vi "VVERFT.vi"(1 "Vector":dbl[](array[numeric])) -> (0 "Funcion de transferencia":string)   [LabVIEW 2019]
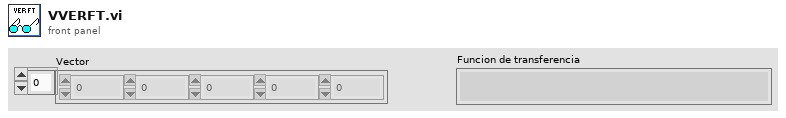
[diagram p1: front panel]
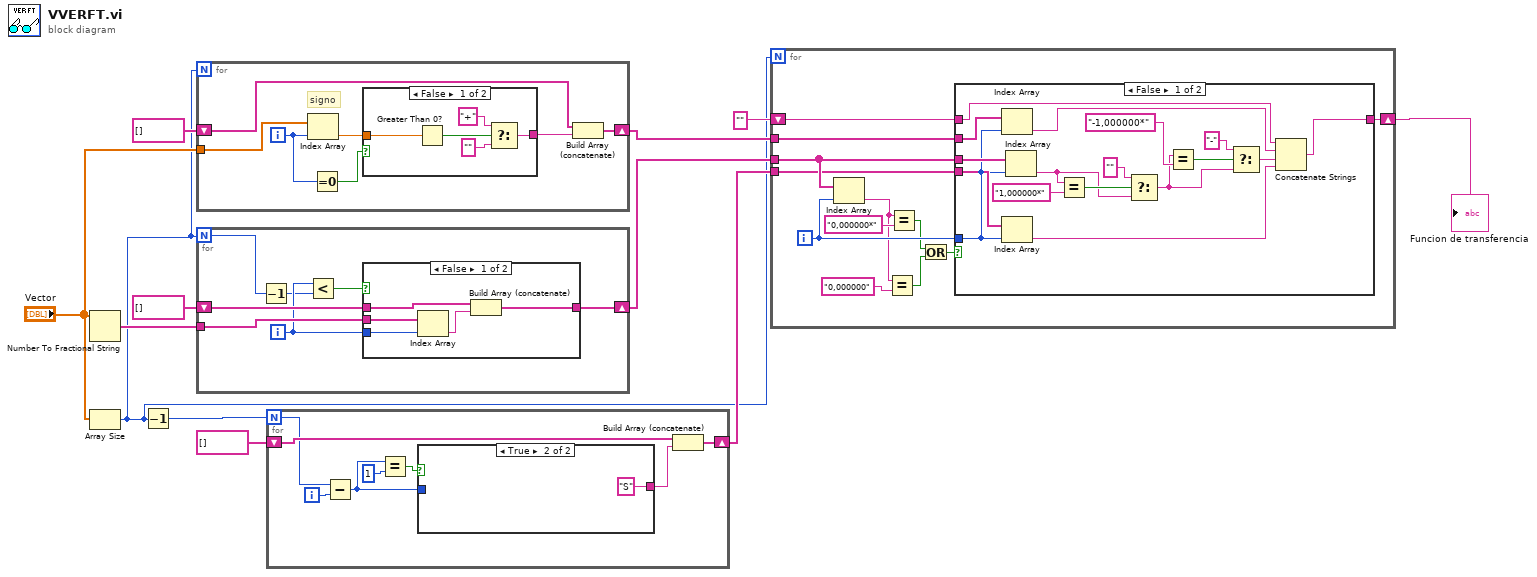
[diagram p0: block diagram]
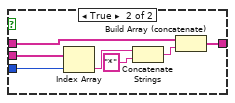
[diagram p2: hidden frame]
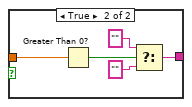
[diagram p4: hidden frame]
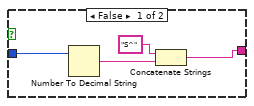
[diagram p5: hidden frame]
diagram:
  n1 = Number To Fractional String(number="Vector") -> (F-format string=w5:string[])  [unwired: 3 in]
  n2 = Array Size(array="Vector") -> (size(s)=w1:i32)
  n3 = Decrement(x=w1) -> (x-1=w2:i32)
  n4 = for {
    N: w1 -> [_]
    tunnel: "Vector" -> [w19]
    shift-right: [w15] -> w10
    shift-left: string[] [] -> [w13]
    i -> [w18]
    # "signo"
    n5 = Index Array(array=w19, index=w18) -> (element=w17:dbl)
    n6 = Equal To 0?(x=w18) -> (x = 0?=w16:bool)
    n7 = case shown="False" w16 {
      tunnel: w17 -> [w20 w28]
      tunnel: [w21 w25] -> w14
      frame False {
        n8 = Greater Than 0?(x=w20) -> (x > 0?=w24:bool)
        n9 = Select(t="+", s=w24, f="") -> (s? t:f=w21:string)
      }
      frame True {
        n10 = Greater Than 0?(x=w28) -> (x > 0?=w29:bool)
        n11 = Select(t="", s=w29, f="") -> (s? t:f=w25:string)
      }
    }
    n12 = Build Array (concatenate)(w13, w14) -> (w15:string[])
  }
  n13 = for {
    N: w1 -> [w31]
    tunnel: w5 -> [w36]
    shift-right: [w34] -> w4
    shift-left: string[] [] -> [w35]
    i -> [w32]
    n14 = Decrement(x=w31) -> (x-1=w30:i32)
    n15 = Less?(x=w32, y=w30) -> (x < y?=w33:bool)
    n16 = case shown="False" w33 {
      tunnel: w36 -> [w39 w48]
      tunnel: w35 -> [w40 w44]
      tunnel: [w41 w43] -> w34
      tunnel: w32 -> [w37 w42]
      frame False {
        n17 = Index Array(array=w39, index=w37) -> (element=w38:string)
        n18 = Build Array (concatenate)(w40, w38) -> (w41:string[])
      }
      frame True {
        n19 = Index Array(array=w48, index=w42) -> (element=w47:string)
        n20 = Concatenate Strings(w47, "*" ("string")) -> (w45:string)
        n21 = Build Array (concatenate)(w44, w45) -> (w43:string[])
      }
    }
  }
  n22 = for {
    N: w2 -> [w49]
    shift-right: [w55] -> w9
    shift-left: string[] [] -> [w54]
    i -> [w56]
    n23 = Subtract(x=w49, y=w56) -> (x-y=w50:i32)
    n24 = Equal?(x=w50, y=1) -> (x = y?=w51:bool)
    n25 = case shown="True" w51 {
      tunnel: [w57 "S" ("string")] -> w53
      tunnel: w50 -> [w58 _]
      frame False {
        n26 = Number To Decimal String(number=w58) -> (decimal integer string=w59:string)  [unwired: 1 in]
        n27 = Concatenate Strings("S^" ("string"), w59) -> (w57:string)
      }
      frame True {
      }
    }
    n28 = Build Array (concatenate)(w54, w53) -> (w55:string[])
  }
  n29 = for {
    N: w1 -> [_]
    tunnel: w4 -> [w71]
    tunnel: w10 -> [w72]
    tunnel: w9 -> [w70]
    shift-right: [w68] -> w8
    shift-left: "" -> [w69]
    i -> [w67]
    n30 = Index Array(array=w71, index=w67) -> (element=w65:string)
    n31 = Equal?(x=w65, y="0,000000") -> (x = y?=w62:bool)
    n32 = Equal?(x=w65, y="0,000000*") -> (x = y?=w63:bool)
    n33 = Or(x=w63, y=w62) -> (x .or. y?=w64:bool)
    n34 = case shown="False" w64 {
      tunnel: w72 -> [w90 _]
      tunnel: w67 -> [w74 _]
      tunnel: w71 -> [w84 _]
      tunnel: w70 -> [w89 _]
      tunnel: w69 -> [w88 w91]
      tunnel: [w87 w91] -> w68
      frame False {
        n35 = Index Array(array=w90, index=w74) -> (element=w86:string)
        n36 = Index Array(array=w89, index=w74) -> (element=w83:string)
        n37 = Index Array(array=w84, index=w74) -> (element=w80:string)
        n38 = Equal?(x=w80, y="1,000000*") -> (x = y?=w82:bool)
        n39 = Select(t="", s=w82, f=w80) -> (s? t:f=w76:string)
        n40 = Equal?(x=w76, y="-1,000000*") -> (x = y?=w78:bool)
        n41 = Select(t="-", s=w78, f=w76) -> (s? t:f=w75:string)
        n42 = Concatenate Strings(w88, w86, w75, w83) -> (w87:string)
      }
      frame True {
      }
    }
  }
  "Funcion de transferencia" <- w8
